vi "Read Panel from INI.vi"(8 "error in (no error)":errorcluster, 10 "VI ref":refnum<vi>, 11 "refnum":T1) -> (0 "error out":errorcluster, 3 "refnum out":T1)   [LabVIEW 2020]
doc: "Read the values of the controls on the Front Panel of <B>VI ref</B> from a standard LabVIEW configuration (INI) file.\n\nUse this VI in conjunction with the <B>Write Panel to INI</B> from the OpenG Variant Config palette."
uses:
  <vilib>/Utility/config.llb/Config Data RefNum.ctl
  <vilib>/Utility/config.llb/NI_LVConfig.lvlib
panel:
  # "Read Panel from INI.vi\n\nReads all Front Panel data from INI file.\n\nPlease visit http://www.OpenG.org to learn about the\nOpen Source LabVIEW software movement.\n\nNOTICE -- YOU MUST LEAVE THIS NOTICE IN PLACE.  PER THE TERMS OF THE LICENSE BELOW, YOU MAY SUBLICENSE THIS SOFTWARE \nIN ANY WAY THAT DOES NOT CONFLICT WITH THIS LICENSE.\n\n### BSD License (http://www.opensource.org/licenses/bsd-license.php) Begin ###\n \nCopyright (c) 2002, Jean-Pierre Drolet <drolet_jp@hotmail.com>\n\nAll rights reserved.\n\nRedistribution and use in source and binary forms, with or without modification, are permitted provided that the following conditions are met:\n\n    * Redistributions of source code must retain the above copyright notice, this list of conditions and the following disclaimer.\n    * Redistributions in binary form must reproduce the above copyright notice, this list of conditions and the following disclaimer in the \n       documentation and/or other materials provided with the distribution.\n    * Neither the name of SciWare, James Kring, Inc., nor the names of its contributors may be used to endorse or promote products derived \n       from this software without specific prior written permission.\n\nTHIS SOFTWARE IS PROVIDED BY THE COPYRIGHT HOLDERS AND CONTRIBUTORS \"AS IS\" AND ANY EXPRESS OR IMPLIED WARRANTIES, \nINCLUDING, BUT NOT LIMITED TO, THE IMPLIED WARRANTIES OF MERCHANTABILITY AND FITNESS FOR A PARTICULAR PURPOSE ARE \nDISCLAIMED. IN NO EVENT SHALL THE COPYRIGHT OWNER OR CONTRIBUTORS BE LIABLE FOR ANY DIRECT, INDIRECT, INCIDENTAL,\n SPECIAL, EXEMPLARY, OR CONSEQUENTIAL DAMAGES (INCLUDING, BUT NOT LIMITED TO, PROCUREMENT OF SUBSTITUTE GOODS OR \nSERVICES; LOSS OF USE, DATA, OR PROFITS; OR BUSINESS INTERRUPTION) HOWEVER CAUSED AND ON ANY THEORY OF LIABILITY, \nWHETHER IN CONTRACT, STRICT LIABILITY, OR TORT (INCLUDING NEGLIGENCE OR OTHERWISE) ARISING IN ANY WAY OUT OF THE USE \nOF THIS SOFTWARE, EVEN IF ADVISED OF THE POSSIBILITY OF SUCH DAMAGE.\n\n### BSD License End ###"
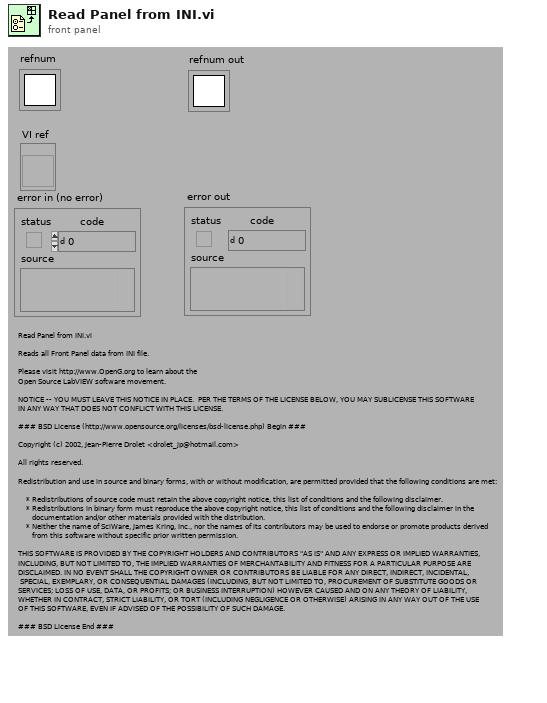
[diagram p1: front panel]
types:
  T1 = typedef "NI_LVConfig.lvlib/Config Data RefNum.ctl" = refnum<k1>
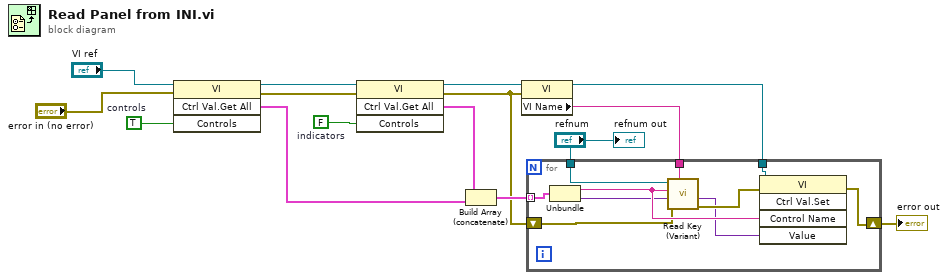
[diagram p0: block diagram]
diagram:
  w13 = FALSE  # indicators
  w15 = TRUE  # controls
  n1 = invoke class="VI" method="Ctrl Val.Get All"(reference="VI ref", error in="error in (no error)", "Controls"=w15) -> (reference out=w14:refnum<vi>, error out=w9:errorcluster, "Get All Control Values Variant"=w11:cluster{"Name":string, "Variant Data":variant}[])  [unwired: 1 in, 1 out]
  n2 = invoke class="VI" method="Ctrl Val.Get All"(reference=w14, error in=w9, "Controls"=w13) -> (reference out=w10:refnum<vi>, error out=w4:errorcluster, "Get All Control Values Variant"=w12:cluster{"Name":string, "Variant Data":variant}[])  [unwired: 1 in, 1 out]
  n3 = Build Array (concatenate)(w12, w11) -> (w8:cluster{"Name":string, "Variant Data":variant}[])
  n4 = property class="VI"(reference=w10, error in=w4) -> (reference out=w1:refnum<vi>, "VI Name"=w7:string)  [unwired: 1 out]
  n5 = for {
    tunnel: w8 -> [w25] mode=indexing
    tunnel: w7 -> [w24]
    tunnel: "refnum" -> [w23]
    shift-right: [w21] -> w3
    shift-left: w4 -> [w17]
    tunnel: w1 -> [w22]
    n6 = Unbundle(w25) -> ("Name"=w19:string, "Variant Data"=w18:variant)
    n7 = call "Read Key (Variant).vi"("section"=w24, "error in (no error)"=w17, "type"=w18, "key (optional)"=w19, "refnum"=w23) -> ("error out"=w20:errorcluster, "key-value"=w16:variant)  [unwired: 3 in, 2 out]
    n8 = invoke class="VI" method="Ctrl Val.Set"(reference=w22, error in=w20, "Control Name"=w19, "Value"=w16) -> (error out=w21:errorcluster)  [unwired: 1 in, 4 out]
  }
  "error out" <- w3
  "refnum out" <- "refnum"
